vi "commTest_3614.vi"() -> ()   [LabVIEW 2012]
panel:
  in  "停止 2":bool
  out "数值 2":i32
  out "错误输出":errorcluster
  out "data out":string
  out "数值":i32
  out "error out":errorcluster caption="错误输出"
  out "remote address":string caption="远程地址"
  out "remote port":u16 caption="远程端口"
  in  "停止":bool
  out "out":string
  in  "in":string
  in  "布尔":bool
  in  "Msg":T1
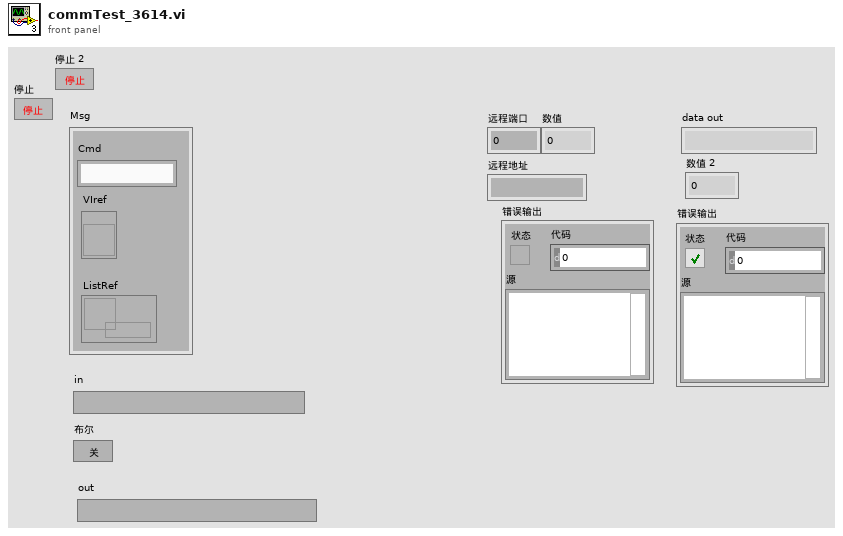
[diagram p1: front panel]
types:
  T1 = cluster{"Cmd":string, "VIref":refnum<vi>, "ListRef":refnum<queue>}
  T2 = enum16{"Standard", "Buffered", "CRLF", "Immediate"}
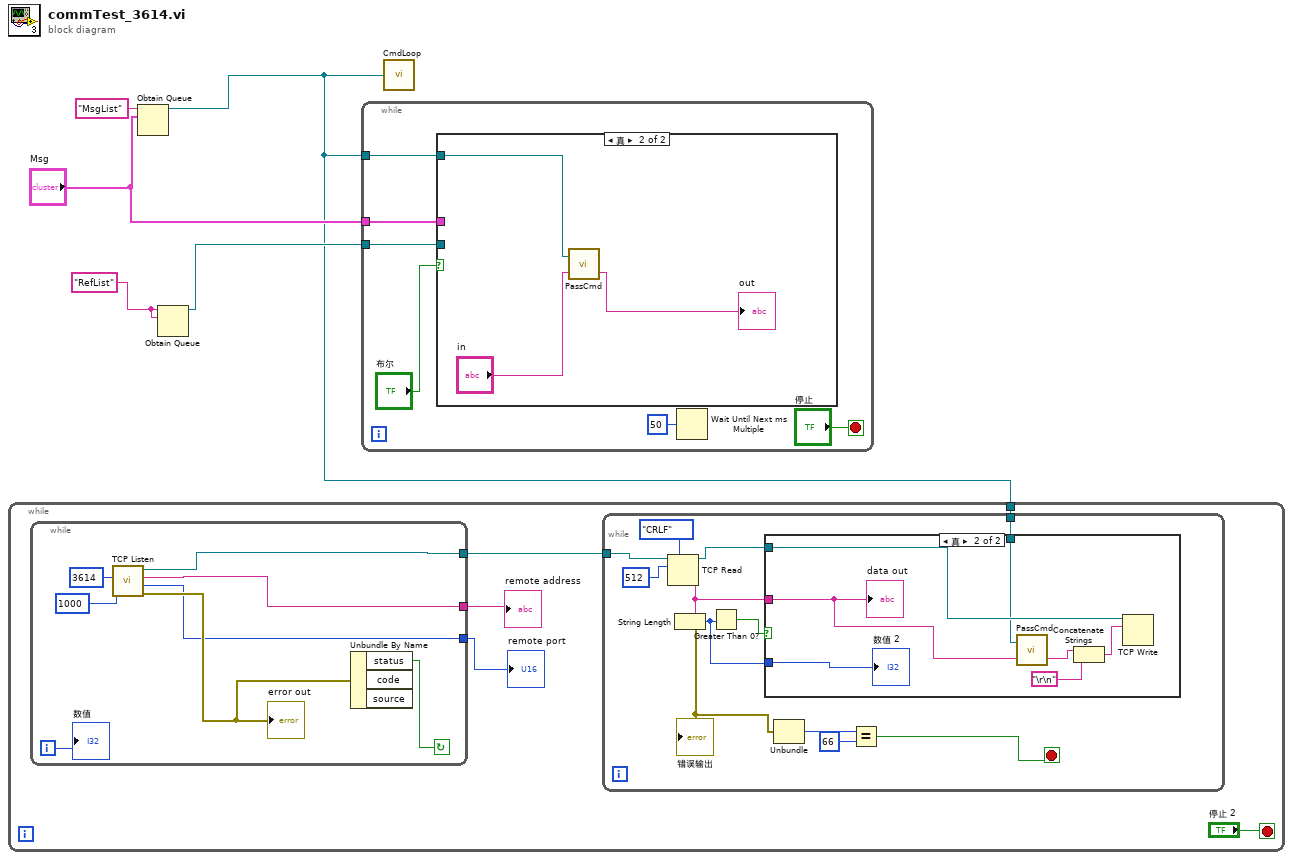
[diagram p0: block diagram]
diagram:
  w4 = "RefList" ("名称（未命名）")
  n1 = Obtain Queue(name (unnamed)="MsgList" ("名称（未命名）"), element data type="Msg") -> (queue out=w1:refnum<queue>)  [unwired: 3 in, 2 out]
  n2 = while {
    tunnel: w1 -> [w7]
    stop <- "停止 2" stop-if-true
    n3 = while {
      tunnel: [w35] -> w8
      tunnel: [w32] -> w10
      tunnel: [w31] -> w9
      i -> [w30]
      stop <- w33 continue-if-true
      n4 = call <vilib>:"TCP Listen.vi"("timeout ms (wait forever: -1)"=1000, "port"=u16 3614) -> ("error out"=w34:errorcluster, "remote port"=w31:u16, "remote address"=w32:string, "connection ID"=w35:refnum<k5>)  [unwired: 5 in, 1 out]
      "error out" <- w34
      n5 = Unbundle By Name(w34) -> ("status"=w33:bool)  [unwired: 2 out]
      "数值" <- w30
    }
    "remote address" <- w10
    "remote port" <- w9
    n6 = while {
      tunnel: w8 -> [w13]
      tunnel: w7 -> [w11]
      stop <- w15 stop-if-true
      n7 = TCP Read(connection ID=w13, bytes to read=512 ("读取的字节"), 7:T2."CRLF" ("模式（标准）")) -> (connection ID out=w12:refnum<k5>, data out=w19:string, error out=w18:errorcluster)  [unwired: 2 in]
      "错误输出" <- w18
      n8 = String Length(string=w19) -> (length=w14:i32)
      n9 = Greater Than 0?(x=w14) -> (x > 0?=w20:bool)
      n10 = case shown="真" w20 {
        tunnel: w19 -> [_ w27]
        tunnel: w14 -> [_ w29]
        tunnel: w12 -> [_ w28]
        tunnel: w11 -> [_ w26]
        frame False {
        }
        frame True {
          n11 = call "PassCmd.vi"("cmd in"=w27, "list ref"=w26) -> ("cmd out"=w25:string)  [unwired: 1 in]
          n12 = Concatenate Strings(w25, "\r\n") -> (w24:string)
          n13 = TCP Write(connection ID=w28, data in=w24) -> ()  [unwired: 2 in, 3 out]
          "data out" <- w27
          "数值 2" <- w29
        }
      }
      n14 = Unbundle(w18) -> ("code"=w17:i32)  [unwired: 2 out]
      n15 = Equal?(x=w17, y=66) -> (x = y?=w15:bool)
    }
  }
  n16 = Obtain Queue(name (unnamed)=w4, element data type=w4) -> (queue out=w3:refnum<queue>)  [unwired: 3 in, 2 out]
  n17 = while {
    tunnel: w1 -> [w42]
    tunnel: w3 -> [w41]
    tunnel: "Msg" -> [w40]
    stop <- "停止" stop-if-true
    n18 = case shown="真" "布尔" {
      tunnel: w42 -> [_ w46]
      tunnel: w41 -> [_ _]
      tunnel: w40 -> [_ _]
      frame False {
      }
      frame True {
        n19 = call "PassCmd.vi"("cmd in"="in", "list ref"=w46) -> ("cmd out"=→"out":string)  [unwired: 1 in]
      }
    }
    n20 = Wait Until Next ms Multiple(millisecond multiple=u32 50 ("毫秒倍数")) -> ()  [unwired: 1 out]
  }
  n21 = call "CmdLoop.vi"("ListRef"=w1) -> ()  [unwired: 1 out]
